vi "Send Error Message.vi"(8 "error in":errorcluster, 9 "Person Reporting":string, 10 "Program Location":string, 11 "Error Code":string) -> (0 "error out":errorcluster)   [LabVIEW 2018, in "MainVIs.lvlib"]
uses:
  MainVIs.lvlib
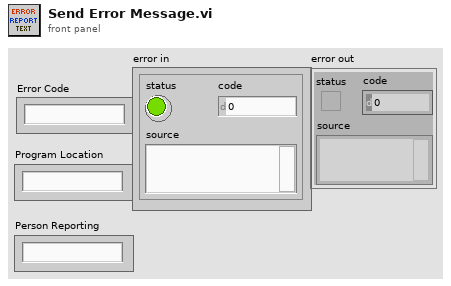
[diagram p1: front panel]
types:
  T1 = enum16{"open", "replace", "create", "open or create", "replace or create", "replace or create with confirmation"}
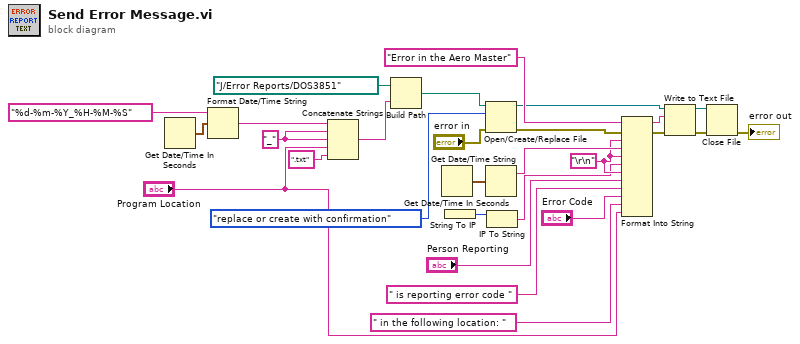
[diagram p0: block diagram]
diagram:
  w5 = "_" ("string")
  w13 = "\r\n"
  n1 = Get Date/Time In Seconds() -> (seconds since 1Jan1904=w7:timestamp)
  n2 = Format Date/Time String(time format string (%c)="%d-%m-%Y_%H-%M-%S", seconds (now)=w7) -> (date/time string=w6:string)  [unwired: 1 in]
  n3 = Concatenate Strings(w6, w5, w5, "Program Location", ".txt" ("string")) -> (w24:string)
  n4 = Build Path(base path=path "J:/Error Reports/DOS3851" ("file path (use dialog)"), name or relative path=w24) -> (appended path=w23:path)
  n5 = Get Date/Time In Seconds() -> (seconds since 1Jan1904=w15:timestamp)
  n6 = String To IP() -> (0:w16:u32)  [unwired: 1 in]
  n7 = Open/Create/Replace File(file path (use dialog)=w23, error in="error in", operation (0:open)=T1."replace or create with confirmation") -> (refnum out=w21:refnum<file>, error out=w17:errorcluster)  [unwired: 3 in, 1 out]
  n8 = Get Date/Time String(seconds (now)=w15) -> (date string=w14:string)  [unwired: 2 in, 1 out]
  n9 = IP To String(2:w16) -> (0:w8:string)  [unwired: 1 in]
  n10 = Format Into String(initial string="Error in the Aero Master", error in=w17, w13, w14, w13, w8, w13, "Person Reporting", " is reporting error code ", "Error Code", " in the following location: " ("input 4"), "Program Location") -> (resulting string=w19:string, error out=w18:errorcluster)  [unwired: 1 in]
  n11 = Write to Text File(file (use dialog)=w21, text=w19, error in=w18) -> (refnum out=w25:refnum<file>, error out=w26:errorcluster)  [unwired: 1 in, 1 out]
  n12 = Close File(refnum=w25, error in=w26) -> (error out=→"error out":errorcluster)  [unwired: 1 out]
